vi "Pachube Get Feed LaunchPad.vi"(7 "timeout ms (60000)":i32=60000, 8 "error in (no error)":errorcluster, 9 "Pachube API Key":string, 10 "Pachube feed ID":string) -> (0 "error out":errorcluster, 1 "Error code":i32, 2 "Error":bool, 3 "Data":string)   [LabVIEW 2010]
doc: "Example of using standard HTTP GET method with LabVIEW TCP/IP vi's to retrieve live data from a Pachube feed. Accessing live feeds need authorisation via an API key which you can request from www.pachube.com.\n\nPachube is a service that enables you to connect, tag and share real time sensor data from objects, devices, buildings and environments around the world. The key aim is to facilitate interaction between remote environments, both physical and virtual. Check out the details of the service at www.pachube.com\n\nThis vi is was created by modifying Bjornar Svingen's Twitter Update Status vi (bjornar.svingen@sintef.no bjornar.svingen@ktv.no).\n\nTo access the Pachube service (which is still beta) you will need an invitation and an API Key - which you can request on the site.\n\nYou can retrive data as either CSV or EEML\n\n EEML is an XML formatted data format which allows you to include meta data such as item names. See www.eeml.org for examples. A simple exmple is shown below:\n \n<?xml version=\"1.0\" encoding=\"UTF-8\"?>\n<eeml xmlns=\"http://www.eeml.org/xsd/005\">\n <environment>\n <data id=\"0\">\n <tag>Power</tag>\n <value>1000</value>\n <unit symbol=\"W\" type=\"derivedSI\">watt</unit>\n </data>\n <data id=\"1\">\n <tag>Temperature</tag>\n <value>21.5</value>\n <unit symbol=\"C\" type=\"derivedSI\">degrees Celsius</unit>\n </data>\n </environment>\n</eeml>\n\n\nIan Bell\nian.bell@ni.com"
panel:
  in  "Duration":string
  in  "Start":timestamp
  in  "Format":string(combo)
  in  "Pachube datastream ID":string="0"
  out "resulting string":string
  out "HTML source":string caption="HTTP response"
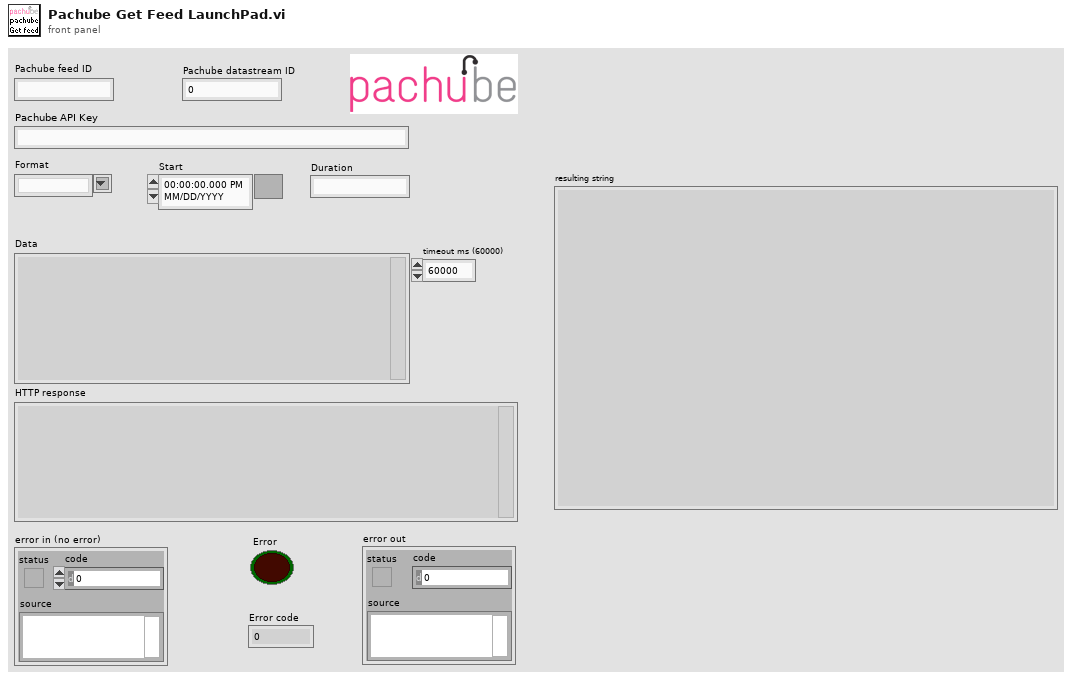
[diagram p1: front panel]
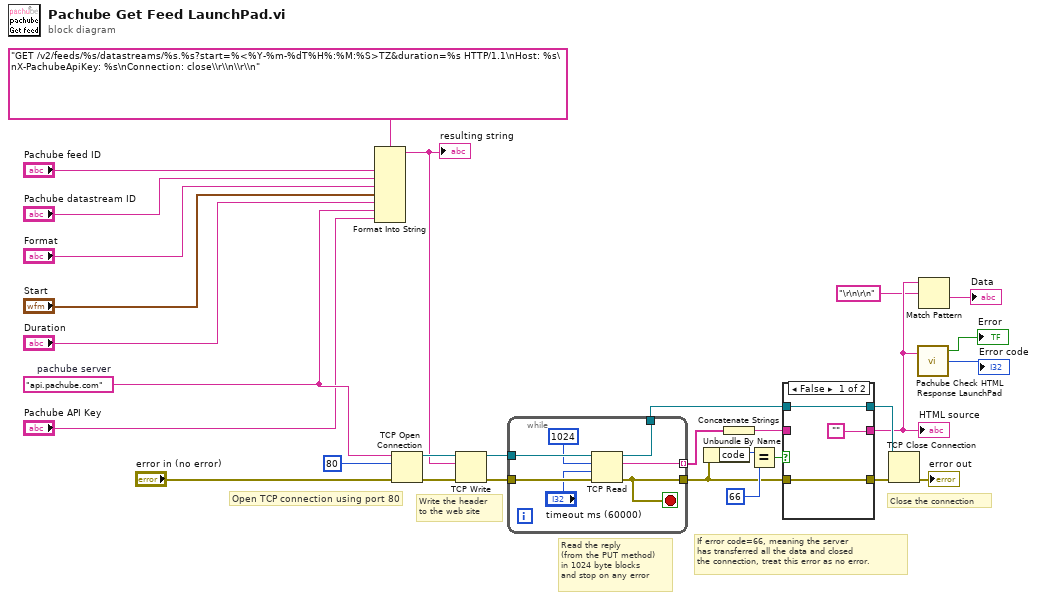
[diagram p0: block diagram]
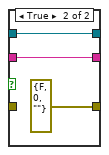
[diagram p2: hidden frame]
diagram:
  w5 = "api.pachube.com"  # pachube server
  # "Close the connection"
  # "If error code=66, meaning the server\nhas transferred all the data and closed\nthe connection, treat this error as no error."
  # "Read the reply\n(from the PUT method)\nin 1024 byte blocks\nand stop on any error"
  # "Write the header\nto the web site"
  # "Open TCP connection using port 80"
  n1 = Format Into String(format string="GET /v2/feeds/%s/datastreams/%s.%s?start=%<%Y-%m-%dT%H%:%M:%S>TZ&duration=%s HTTP/1.1\nHost: %s\nX-PachubeApiKey: %s\nConnection: close\\r\\n\\r\\n" ("Command"), "Pachube feed ID", "Pachube datastream ID", "Format", "Start", "Duration", w5, "Pachube API Key") -> (resulting string=w3:string)  [unwired: 2 in, 1 out]
  "resulting string" <- w3
  n2 = TCP Open Connection(address=w5, remote port or service name=u16 80 ("remote port"), error in (no error)="error in (no error)") -> (connection ID=w27:refnum<k5>, error out=w28:errorcluster)  [unwired: 2 out]
  n3 = TCP Write(connection ID=w27, data in=w3, error in (no error)=w28) -> (connection ID out=w24:refnum<k5>, error out=w23:errorcluster)  [unwired: 2 out]
  n4 = while {
    tunnel: w23 -> [w37]
    tunnel: w24 -> [w36]
    tunnel: [w32] -> w21
    tunnel: [w35] -> w18
    tunnel: [w34] -> w20 mode=indexing
    stop <- w32 stop-if-true
    n5 = TCP Read(connection ID=w36, bytes to read=1024, error in (no error)=w37, 9:"timeout ms (60000)") -> (connection ID out=w35:refnum<k5>, data out=w34:string, error out=w32:errorcluster)  [unwired: 1 out]
  }
  n6 = Unbundle By Name(w21) -> ("code"=w26:i32)
  n7 = Concatenate Strings(w20) -> (w19:string)
  n8 = Equal?(x=w26, y=66) -> (x = y?=w25:bool)
  n9 = case shown="False" w25 {
    tunnel: ["" w42] -> w12
    tunnel: w19 -> [_ w42]
    tunnel: [w39 errorcluster {"status"=FALSE, "code"=0, "source"=""} ("error in (no error)")] -> w16
    tunnel: w21 -> [w39 _]
    tunnel: w18 -> [w38 w41]
    tunnel: [w38 w41] -> w17
    frame False {
    }
    frame True {
    }
  }
  "HTML source" <- w12
  n10 = TCP Close Connection(connection ID=w17, error in (no error)=w16) -> (error out=→"error out":errorcluster)  [unwired: 2 out]
  n11 = call "Pachube Check HTML Response LaunchPad.vi"("HTML Response"=w12) -> ("Error"=→"Error":bool, "Error code"=→"Error code":i32)  [unwired: 1 in, 1 out]
  n12 = Match Pattern(string=w12, regular expression="\r\n\r\n") -> (after substring=→"Data":string)  [unwired: 4 out]
